vi "GetTaskType.vi"(2 "Task Path":string) -> (0 "task type":i32, 1 "task path":string)   [LabVIEW 2009]
uses:
  Windows/System32/AdvLvDaq.dll
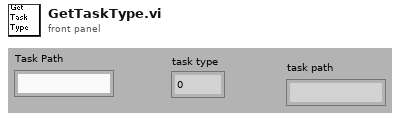
[diagram p1: front panel]
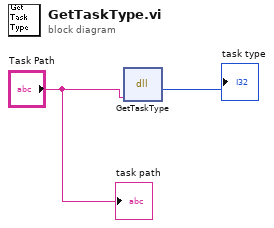
[diagram p0: block diagram]
diagram:
  n1 = dll-call lib="C:/Windows/System32/AdvLvDaq.dll" fn="GetTaskType"("taskPath"="Task Path") -> ("return type"=→"task type":i32)  [unwired: 3 in, 3 out]
  "task path" <- "Task Path"
